vi "Exercise1.19-Real Time Display.vi"() -> ()   [LabVIEW 2013]
panel:
  out "Waveform Chart":cluster{"number: 0 to 1":dbl, dbl}(graph)
  out "Waveform Chart":dbl(graph)
  in  "stop 2":bool
  in  "stop":bool
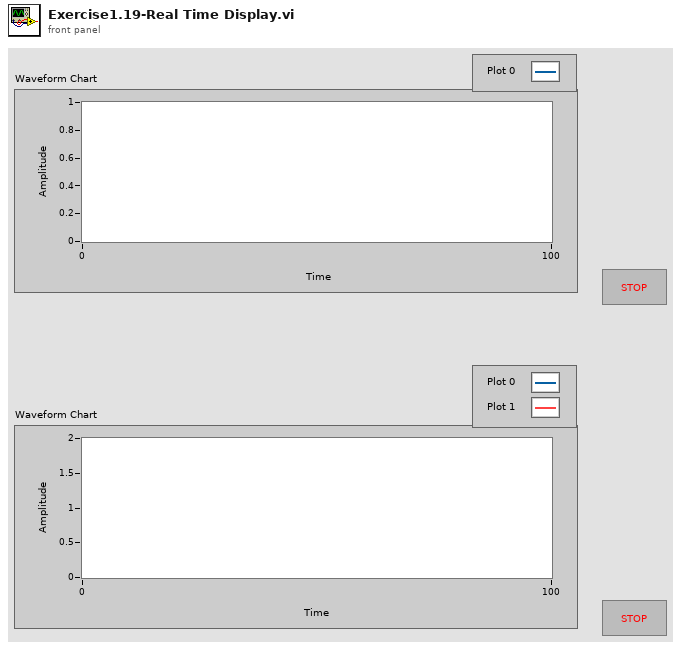
[diagram p1: front panel]
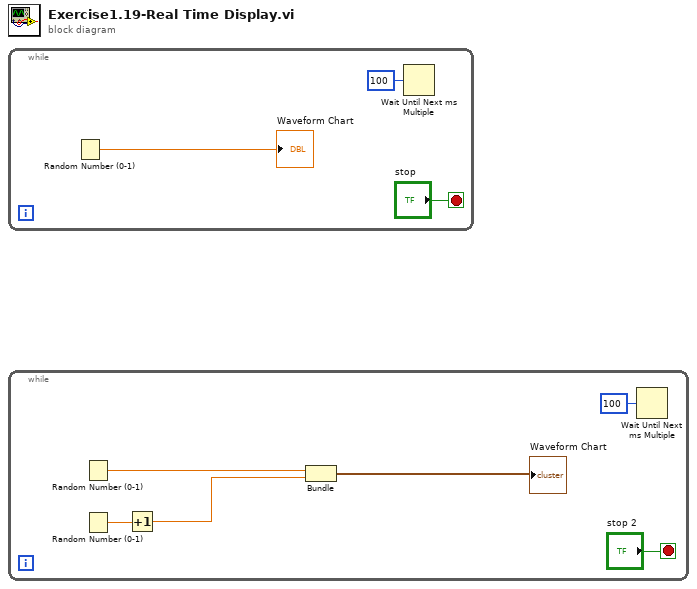
[diagram p0: block diagram]
diagram:
  n1 = while {
    stop <- "stop" stop-if-true
    n2 = Random Number (0-1)() -> (number: 0 to 1=→"Waveform Chart":dbl)
    n3 = Wait Until Next ms Multiple(millisecond multiple=u32 100) -> ()  [unwired: 1 out]
  }
  n4 = while {
    stop <- "stop 2" stop-if-true
    n5 = Random Number (0-1)() -> (number: 0 to 1=w7:dbl)
    n6 = Random Number (0-1)() -> (number: 0 to 1=w6:dbl)
    n7 = Increment(x=w6) -> (x+1=w5:dbl)
    n8 = Bundle "Bundle"("number: 0 to 1"=w7, w5) -> (→"Waveform Chart":cluster{"number: 0 to 1":dbl, dbl})  [unwired: 1 in]
    n9 = Wait Until Next ms Multiple(millisecond multiple=u32 100) -> ()  [unwired: 1 out]
  }
